vi "ExportPicture.vi"(1 "Palette Number (gray)":T2(ring), 3 "16bit Image?":bool, 4 "Image":T1, 5 "Image Scalebar":T1, 6 "name input":string, 7 "Path":refnum<vi>, 8 "notes 2":refnum<vi>) -> (0 "Numeric":i32, 2 "error out":errorcluster)   [LabVIEW 2009]
uses:
  <vilib>/vision/Image Controls.llb/IMAQ Image.ctl
panel:
  out "String 2":string
  in  "autosave":bool
  in  "cancel":bool
  in  "Save":bool
  in  "File Path":path
  in  "Image Quality":u32=750 max=1000 step=10
  in  "Compress BMP?":bool
  in  "Data type":u16(ring) items=["Windows Bitmap", "JPG", "TIFF", "PNG"]
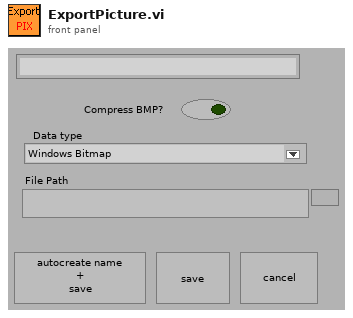
[diagram p1: front panel]
types:
  T1 = typedef "IMAQ Image.ctl" = refnum<image>
  T2 = enum32{"Gray", "Binary", "Gradient", "Rainbow", "Temperature"}
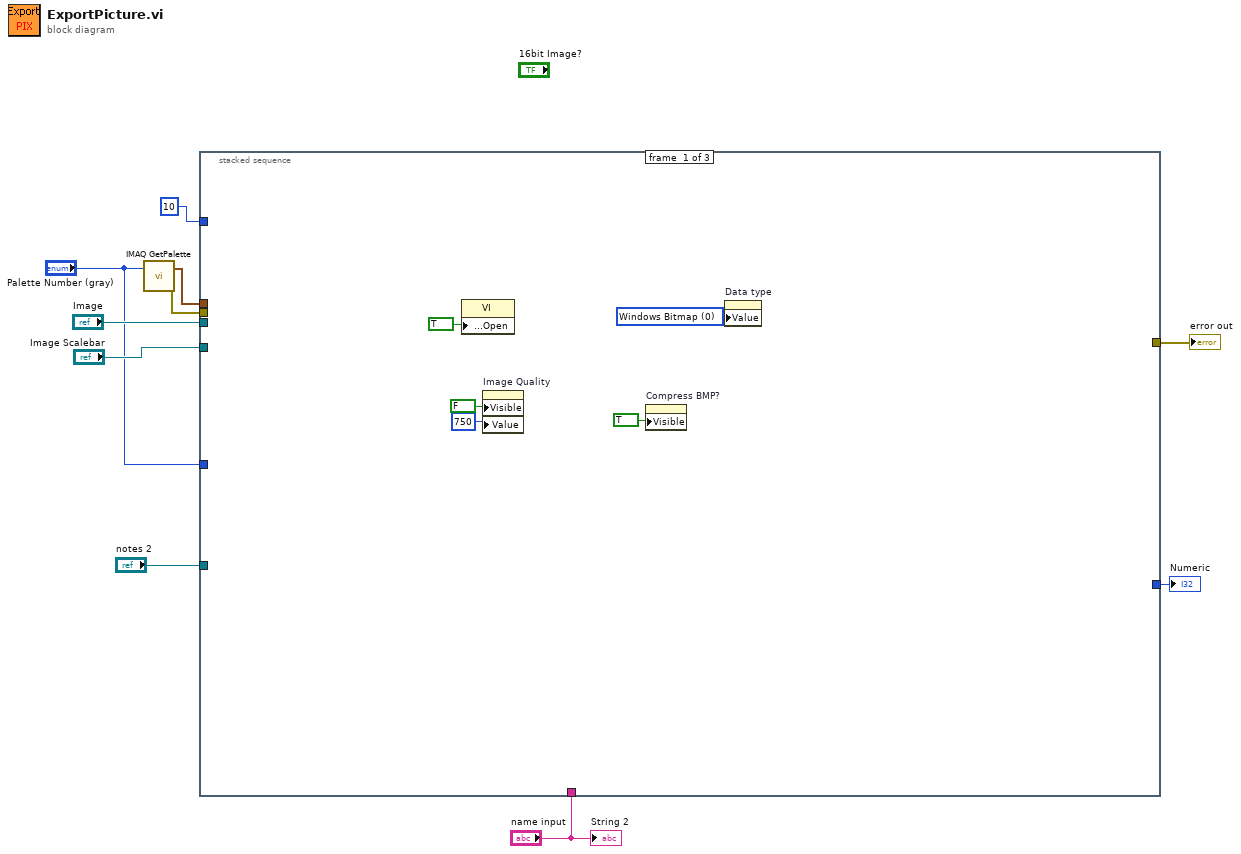
[diagram p0: block diagram]
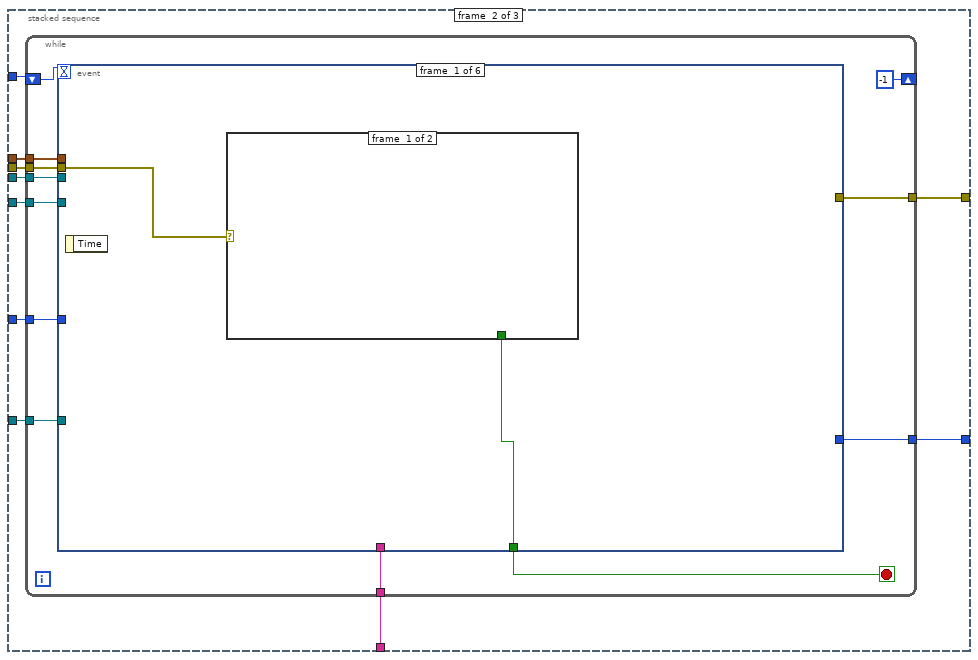
[diagram p2: hidden frame]
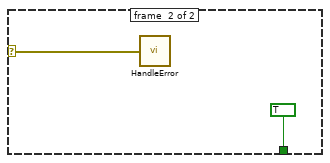
[diagram p3: hidden frame]
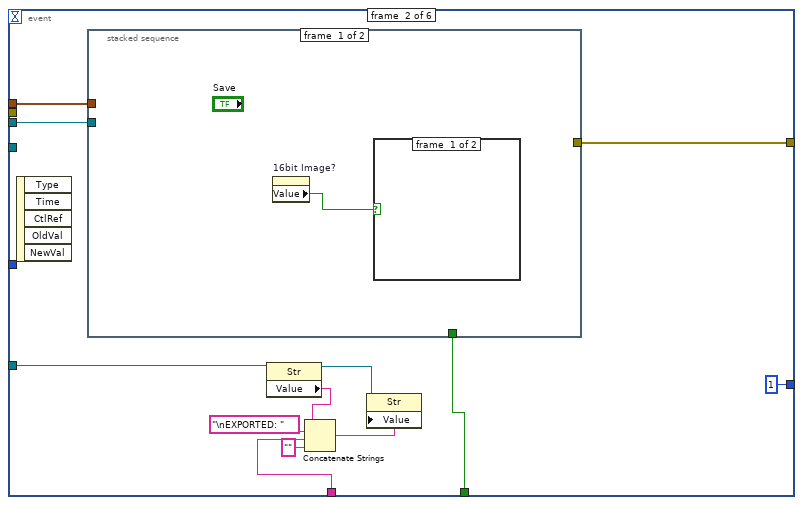
[diagram p4: hidden frame]
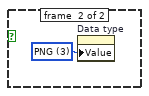
[diagram p5: hidden frame]
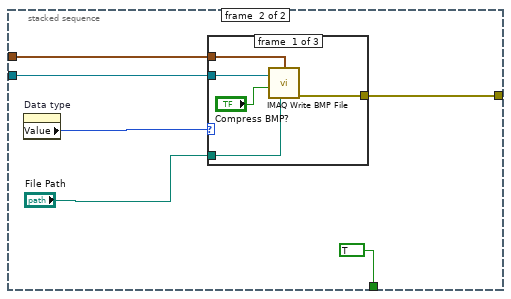
[diagram p6: hidden frame]
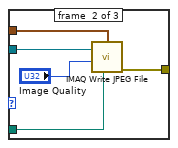
[diagram p7: hidden frame]
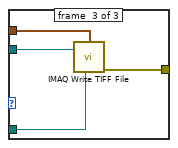
[diagram p8: hidden frame]
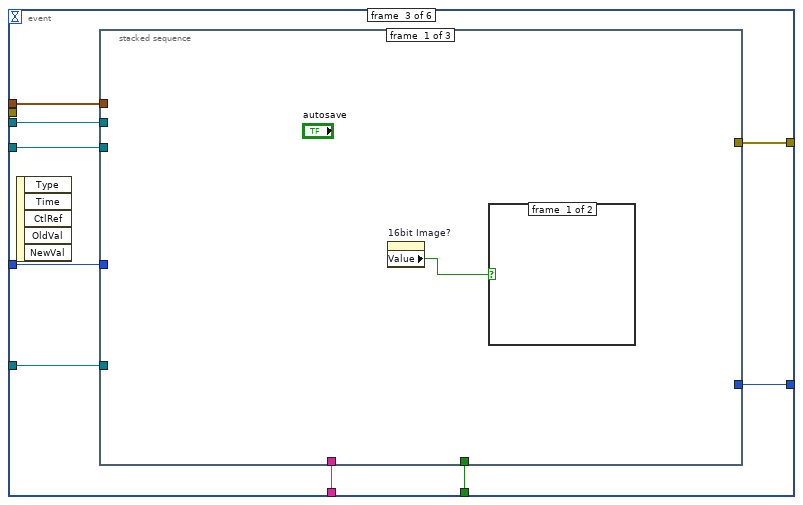
[diagram p9: hidden frame]
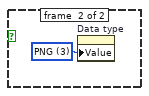
[diagram p10: hidden frame]
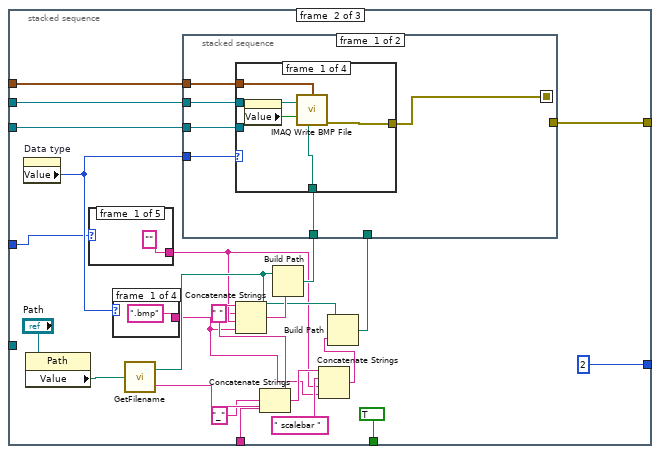
[diagram p11: hidden frame]
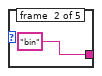
[diagram p12: hidden frame]
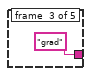
[diagram p13: hidden frame]
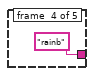
[diagram p14: hidden frame]
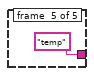
[diagram p15: hidden frame]
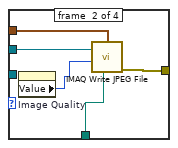
[diagram p16: hidden frame]
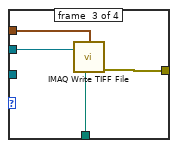
[diagram p17: hidden frame]
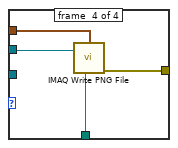
[diagram p18: hidden frame]
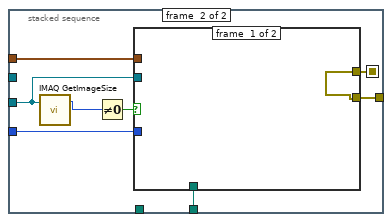
[diagram p19: hidden frame]
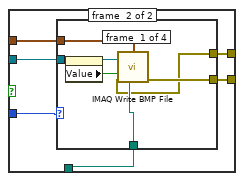
[diagram p20: hidden frame]
diagram:
  n1 = call "IMAQ GetPalette"("Palette Number (gray)"="Palette Number (gray)") -> ("Color Palette"=w7:cluster{"Red":u8, "Green":u8, "Blue":u8}[], "error out"=w6:errorcluster)  [unwired: 4 in]
  n2 = stacked-sequence {
    tunnel: "Image" -> [_ w25 _]
    tunnel: [_ w24 _] -> w10
    tunnel: "name input" -> [_ w23 _]
    tunnel: w7 -> [_ w22 _]
    tunnel: w6 -> [_ w21 _]
    tunnel: 10 -> [_ w20 _]
    tunnel: "Image Scalebar" -> [_ w19 _]
    tunnel: [_ w18 _] -> w3
    tunnel: "Palette Number (gray)" -> [_ w17 _]
    tunnel: "notes 2" -> [_ w16 _]
    frame #0 {
      w11 = u16 0 items=["Windows Bitmap", "JPG", "TIFF"] ("Data type")
      n3 = property class="VI"("Front Panel Window:Open"=TRUE) -> ()  [unwired: 2 in, 2 out]
      n4 = property on="Image Quality" class="Digital (strict)"("Visible"=FALSE, "Value"=u32 750 ("Image Quality")) -> ()  [unwired: 2 in, 2 out]
      n5 = property on="Compress BMP?" class="Boolean (strict)"("Visible"=TRUE) -> ()  [unwired: 2 in, 2 out]
      n6 = property on="Data type" class="Ring (strict)"("Value"=w11) -> ()  [unwired: 2 in, 2 out]
    }
    frame #1 {
      n7 = while {
        tunnel: w25 -> [w37]
        tunnel: [w36] -> w24
        tunnel: w23 -> [w34]
        tunnel: w22 -> [w33]
        tunnel: w21 -> [w32]
        shift-right: [-1] -> _
        shift-left: w20 -> [w31]
        tunnel: w19 -> [w29]
        tunnel: [w28] -> w18
        tunnel: w17 -> [w27]
        tunnel: w16 -> [w26]
        stop <- w35 stop-if-true
        n8 = event shown="[1] \"Save\": Value Change" {
          selector: _ -> [_ _ _ _ _ _]
          dyn-events: _ -> [_ _ _ _ _ _]
          timeout: w31 -> [_ _ _ _ _ _]
          tunnel: w37 -> [_ w53 w84 _ _ _]
          tunnel: [_ w52 w81 _ _ _] -> w36
          tunnel: [w38 w51 w82 _ w196 w199] -> w35
          tunnel: w34 -> [_ w43 w83 _ _ _]
          tunnel: w33 -> [_ w50 w80 _ _ _]
          tunnel: w32 -> [w39 _ _ _ _ _]
          tunnel: w29 -> [_ _ w79 _ _ _]
          tunnel: [_ 1 w78 _ _ _] -> w28
          tunnel: w27 -> [_ _ w77 _ _ _]
          tunnel: w26 -> [_ w42 w76 _ _ _]
          event #0 {
            n9 = event-data() -> ()  [unwired: 1 in, 1 out]
            n10 = case shown="Error" w39 {
              selector: w39 -> [_ w40]
              tunnel: [_ TRUE] -> w38
              frame #0 {
              }
              frame #1 {
                n11 = call "HandleError.vi"("error in (no error)"=w40) -> ()
              }
            }
          }
          event #1 {
            n12 = event-data() -> ()  [unwired: 1 in, 5 out]
            n13 = stacked-sequence {
              tunnel: w53 -> [_ w61]
              tunnel: [_ w60] -> w52
              tunnel: [_ TRUE] -> w51
              tunnel: w50 -> [_ w56]
              frame #0 {
                n14 = property on="16bit Image?" class="Boolean (strict)"() -> ("Value"=w54:bool)  [unwired: 2 in, 2 out]
                n15 = case shown="True" w54 {
                  frame #0 {
                  }
                  frame #1 {
                    w55 = u16 3 items=["Windows Bitmap", "JPG", "TIFF", "PNG"] ("Data type")
                    n16 = property on="Data type" class="Ring (strict)"("Value"=w55) -> ()  [unwired: 2 in, 2 out]
                  }
                }
              }
              frame #1 {
                n17 = property on="Data type" class="Ring (strict)"() -> ("Value"=w59:u16)  [unwired: 2 in, 2 out]
                n18 = case shown="0, Default" w59 {
                  tunnel: "File Path" -> [w64 w69 w75]
                  tunnel: w61 -> [w66 w71 w74]
                  tunnel: [w65 w70 w73] -> w60
                  tunnel: w56 -> [w62 w67 w72]
                  frame #0 {
                    n19 = call "IMAQ Write BMP File"("Compress?"="Compress BMP?", "File Path"=w64, "Image"=w66, "Color Palette"=w62) -> ("error out"=w65:errorcluster)  [unwired: 4 in]
                  }
                  frame #1 {
                    n20 = call "IMAQ Write JPEG File"("Image Quality"="Image Quality", "File Path"=w69, "Image"=w71, "Color Palette"=w67) -> ("error out"=w70:errorcluster)  [unwired: 4 in]
                  }
                  frame #2 {
                    n21 = call "IMAQ Write TIFF File"("File Path"=w75, "Image"=w74, "Color Palette"=w72) -> ("error out"=w73:errorcluster)  [unwired: 5 in]
                  }
                }
              }
            }
            n22 = property class="Str"(reference=w42) -> (reference out=w48:refnum<vi>, "Value"=w47:string)  [unwired: 1 in, 1 out]
            n23 = Concatenate Strings(w47, "\nEXPORTED: " ("string"), w43, "" ("string")) -> (w44:string)
            n24 = property class="Str"(reference=w48, "Value"=w44) -> ()  [unwired: 1 in, 2 out]
          }
          event #2 {
            n25 = event-data() -> ()  [unwired: 1 in, 5 out]
            n26 = stacked-sequence {
              tunnel: w84 -> [_ w109 _]
              tunnel: [_ w108 _] -> w81
              tunnel: [_ TRUE _] -> w82
              tunnel: w83 -> [_ w105 w180]
              tunnel: w80 -> [_ w100 _]
              tunnel: w79 -> [_ w99 _]
              tunnel: [_ 2 _] -> w78
              tunnel: w77 -> [_ w92 _]
              tunnel: w76 -> [_ _ w181]
              frame #0 {
                n27 = property on="16bit Image?" class="Boolean (strict)"() -> ("Value"=w85:bool)  [unwired: 2 in, 2 out]
                n28 = case shown="True" w85 {
                  frame #0 {
                  }
                  frame #1 {
                    w86 = u16 3 items=["Windows Bitmap", "JPG", "TIFF", "PNG"] ("Data type")
                    n29 = property on="Data type" class="Ring (strict)"("Value"=w86) -> ()  [unwired: 2 in, 2 out]
                  }
                }
              }
              frame #1 {
                n30 = property on="Data type" class="Ring (strict)"() -> ("Value"=w104:u16)  [unwired: 2 in, 2 out]
                n31 = property class="Path"(reference="Path") -> ("Value"=w87:path)  [unwired: 1 in, 2 out]
                n32 = case shown="\"Gray\", Default" w92 {
                  tunnel: ["" "bin" "grad" "rainb" "temp"] -> w89
                  frame #0 {
                  }
                  frame #1 {
                  }
                  frame #2 {
                  }
                  frame #3 {
                  }
                  frame #4 {
                  }
                }
                n33 = case shown="3" w104 {
                  tunnel: [".bmp" ".jpg" ".tif" ".png"] -> w90
                  frame #0 {
                  }
                  frame #1 {
                  }
                  frame #2 {
                  }
                  frame #3 {
                  }
                }
                n34 = call "GetFilename.vi"("Value"=w87) -> ("base path"=w96:path, "name"=w102:string)
                n35 = Concatenate Strings(w102, "_" ("string"), w105) -> (w91:string)
                n36 = Concatenate Strings(w91, " " ("string"), w89, w90) -> (w98:string)
                n37 = Build Path(base path=w96, name or relative path=w98) -> (appended path=w103:path)
                n38 = Concatenate Strings(w91, " scalebar " ("string"), w89, w90) -> (w97:string)
                n39 = Build Path(base path=w96, name or relative path=w97) -> (appended path=w94:path)
                n40 = stacked-sequence {
                  seq-local: [w115 _] -> [_ w144]
                  tunnel: w109 -> [w120 _]
                  tunnel: [_ w145] -> w108
                  tunnel: w104 -> [w119 w142]
                  tunnel: w103 -> [w118 _]
                  tunnel: w100 -> [w117 w146]
                  tunnel: w99 -> [w116 w141]
                  tunnel: w94 -> [_ w143]
                  frame #0 {
                    n41 = case shown="3" w119 {
                      tunnel: w118 -> [w123 w128 w134 w135]
                      tunnel: w120 -> [w125 w130 w133 w137]
                      tunnel: [w124 w129 w132 w136] -> w115
                      tunnel: w117 -> [w121 w126 w131 w138]
                      tunnel: w116 -> [_ _ _ _]
                      frame #0 {
                        n42 = property on="Compress BMP?" class="Boolean (strict)"() -> ("Value"=w122:bool)  [unwired: 2 in, 2 out]
                        n43 = call "IMAQ Write BMP File"("Compress?"=w122, "File Path"=w123, "Image"=w125, "Color Palette"=w121) -> ("error out"=w124:errorcluster)  [unwired: 4 in]
                      }
                      frame #1 {
                        n44 = property on="Image Quality" class="Digital (strict)"() -> ("Value"=w127:u32)  [unwired: 2 in, 2 out]
                        n45 = call "IMAQ Write JPEG File"("Image Quality"=w127, "File Path"=w128, "Image"=w130, "Color Palette"=w126) -> ("error out"=w129:errorcluster)  [unwired: 4 in]
                      }
                      frame #2 {
                        n46 = call "IMAQ Write TIFF File"("File Path"=w134, "Image"=w133, "Color Palette"=w131) -> ("error out"=w132:errorcluster)  [unwired: 5 in]
                      }
                      frame #3 {
                        n47 = call "IMAQ Write PNG File"("File Path"=w135, "Image"=w137, "Color Palette"=w138) -> ("error out"=w136:errorcluster)  [unwired: 5 in]
                      }
                    }
                  }
                  frame #1 {
                    n48 = call "IMAQ GetImageSize"("Image"=w141) -> ("Y Resolution"=w139:i32)  [unwired: 3 in, 2 out]
                    n49 = Not Equal To 0?(x=w139) -> (x != 0?=w140:bool)
                    n50 = case shown="False" w140 {
                      tunnel: w146 -> [_ w153]
                      tunnel: w141 -> [_ w152]
                      tunnel: [w147 w151] -> w145
                      tunnel: w144 -> [w147 w150]
                      tunnel: w143 -> [_ w149]
                      tunnel: w142 -> [_ w148]
                      frame #0 {
                      }
                      frame #1 {
                        n51 = case shown="3" w148 {
                          tunnel: w149 -> [w157 w163 w170 w172]
                          tunnel: w152 -> [w159 w165 w169 w174]
                          tunnel: [w158 w164 w168 w171] -> w151
                          tunnel: w153 -> [w155 w161 w167 w175]
                          tunnel: w150 -> [w154 w160 w166 w173]
                          frame #0 {
                            n52 = property on="Compress BMP?" class="Boolean (strict)"() -> ("Value"=w156:bool)  [unwired: 2 in, 2 out]
                            n53 = call "IMAQ Write BMP File"("error in (no error)"=w154, "Compress?"=w156, "File Path"=w157, "Image"=w159, "Color Palette"=w155) -> ("error out"=w158:errorcluster)  [unwired: 3 in]
                          }
                          frame #1 {
                            n54 = property on="Image Quality" class="Digital (strict)"() -> ("Value"=w162:u32)  [unwired: 2 in, 2 out]
                            n55 = call "IMAQ Write JPEG File"("error in (no error)"=w160, "Image Quality"=w162, "File Path"=w163, "Image"=w165, "Color Palette"=w161) -> ("error out"=w164:errorcluster)  [unwired: 3 in]
                          }
                          frame #2 {
                            n56 = call "IMAQ Write TIFF File"("error in (no error)"=w166, "File Path"=w170, "Image"=w169, "Color Palette"=w167) -> ("error out"=w168:errorcluster)  [unwired: 4 in]
                          }
                          frame #3 {
                            n57 = call "IMAQ Write PNG File"("error in (no error)"=w173, "File Path"=w172, "Image"=w174, "Color Palette"=w175) -> ("error out"=w171:errorcluster)  [unwired: 4 in]
                          }
                        }
                      }
                    }
                  }
                }
              }
              frame #2 {
                n58 = property class="Str"(reference=w181) -> (reference out=w182:refnum<vi>, "Value"=w183:string)  [unwired: 1 in, 1 out]
                n59 = Concatenate Strings(w183, "\nEXPORTED: " ("string"), w180, "" ("string")) -> (w186:string)
                n60 = property class="Str"(reference=w182, "Value"=w186) -> ()  [unwired: 1 in, 2 out]
              }
            }
          }
          event #3 {
            n61 = event-data() -> ()  [unwired: 1 in, 5 out]
            n62 = case shown="3" "Data type" {
              frame #0 {
                n63 = property on="Compress BMP?" class="Boolean (strict)"("Visible"=TRUE) -> ()  [unwired: 2 in, 2 out]
                n64 = property on="Image Quality" class="Digital (strict)"("Visible"=FALSE) -> ()  [unwired: 2 in, 2 out]
              }
              frame #1 {
                n65 = property on="Compress BMP?" class="Boolean (strict)"("Visible"=FALSE) -> ()  [unwired: 2 in, 2 out]
                n66 = property on="Image Quality" class="Digital (strict)"("Visible"=FALSE) -> ()  [unwired: 2 in, 2 out]
              }
              frame #2 {
                n67 = property on="Compress BMP?" class="Boolean (strict)"("Visible"=FALSE) -> ()  [unwired: 2 in, 2 out]
                n68 = property on="Image Quality" class="Digital (strict)"("Visible"=TRUE) -> ()  [unwired: 2 in, 2 out]
              }
              frame #3 {
                n69 = property on="Compress BMP?" class="Boolean (strict)"("Visible"=FALSE) -> ()  [unwired: 2 in, 2 out]
                n70 = property on="Image Quality" class="Digital (strict)"("Visible"=FALSE) -> ()  [unwired: 2 in, 2 out]
              }
            }
          }
          event #4 {
            n71 = event-data() -> ()  [unwired: 1 in, 5 out]
            n72 = stacked-sequence {
              tunnel: [_ TRUE] -> w196
              frame #0 {
              }
              frame #1 {
              }
            }
          }
          event #5 {
            n73 = event-data() -> ()  [unwired: 1 in, 3 out]
            n74 = stacked-sequence {
              tunnel: [w200] -> w199
              frame #0 {
                n75 = Two Button Dialog(message="Quit without saving?") -> (T button?=w200:bool)  [unwired: 2 in]
              }
            }
            n76 = Not(x=w199) -> (.not. x?=w198:bool)
            n77 = event-data("Discard?"=w198) -> ()  [unwired: 1 in, 1 out]
          }
        }
      }
    }
    frame #2 {
      n78 = property class="VI"("Front Panel Window:Open"=FALSE) -> ()  [unwired: 2 in, 2 out]
    }
  }
  "error out" <- w10
  "Numeric" <- w3
  "String 2" <- "name input"
